vi "Microscope.Initialized.vi"(8 "error in (no error)":errorcluster, 10 "Initialized":T1, 11 "Microscope":refnum<class "Microscope.lvclass">) -> (0 "error out":errorcluster, 3 "Microscope out":refnum<class "Microscope.lvclass">)   [LabVIEW 2013, in "Microscope.lvclass"]
doc: "---------------------------------------------------------------\nJKI State Machine Objects™\nhttp://jki.net/state-machine-objects/\nCopyright (C) 2005-2015, JKI <info@jki.net>\nALL RIGHTS RESERVEDJKI State Machine Objects (SMO) 1.0.0.4\nJKI - JKI\nCopyright (c) 2015, JKI"
uses:
  Microscope.lvclass
  Typedefs/PublicEvents--Microscope.Initialized.ctl
panel:
  # "For instructions on how to use the JKI State Machine Objects, examples and video tutorials, visit:\nhttp://jki.net/state-machine-objects/\n\nJKI State Machine Objects™\nhttp://jki.net/state-machine-objects/\nCopyright (C) 2005-2015, JKI <info@jki.net>\nALL RIGHTS RESERVED"
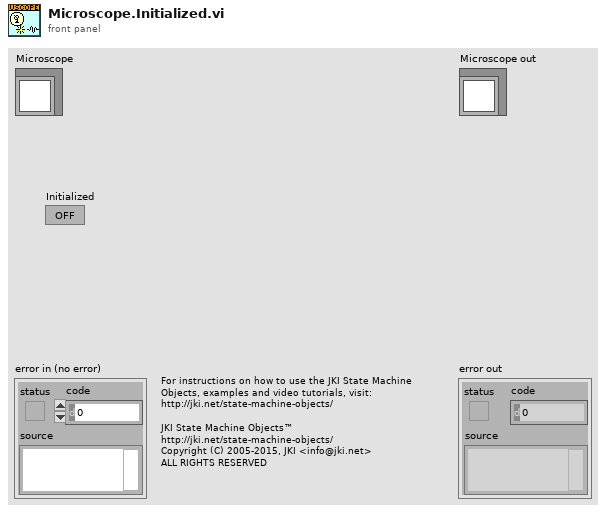
[diagram p1: front panel]
types:
  T1 = typedef "Microscope.lvclass/PublicEvents--Microscope.Initialized.ctl" = bool
  T2 = typedef "Microscope.lvclass/PrivateData--Ref.ctl" = refnum<data-value>
  T3 = typedef "Microscope.lvclass/PrivateData--Cluster.ctl" = cluster{"Public Events":T4, "Protected Events":T5, "Private Events":T6, "Dependencies":T7, "Configuration":T8}
  T4 = typedef "Microscope.lvclass/PublicEvents--Cluster.ctl" = cluster{"Value Changed":refnum<user-event>, "Initialized":refnum<user-event>}
  T5 = typedef "Microscope.lvclass/ProtectedEvents--Cluster.ctl" = cluster{"placeholder":refnum<user-event>}
  T6 = typedef "Microscope.lvclass/PrivateEvents--Cluster.ctl" = cluster{"New Value":refnum<user-event>, "Initialize":refnum<user-event>, "CaptureImageAtPosition":refnum<user-event>}
  T7 = typedef "Microscope.lvclass/Dependencies--Cluster.ctl" = cluster{"XYStage":refnum<class "XYStage.lvclass">, "Camera":refnum<class "Camera.lvclass">}
  T8 = typedef "Microscope.lvclass/Configuration--Cluster.ctl" = cluster{"XY Stage":string, "Camera":string, "image output folder":path, "filetype":string}
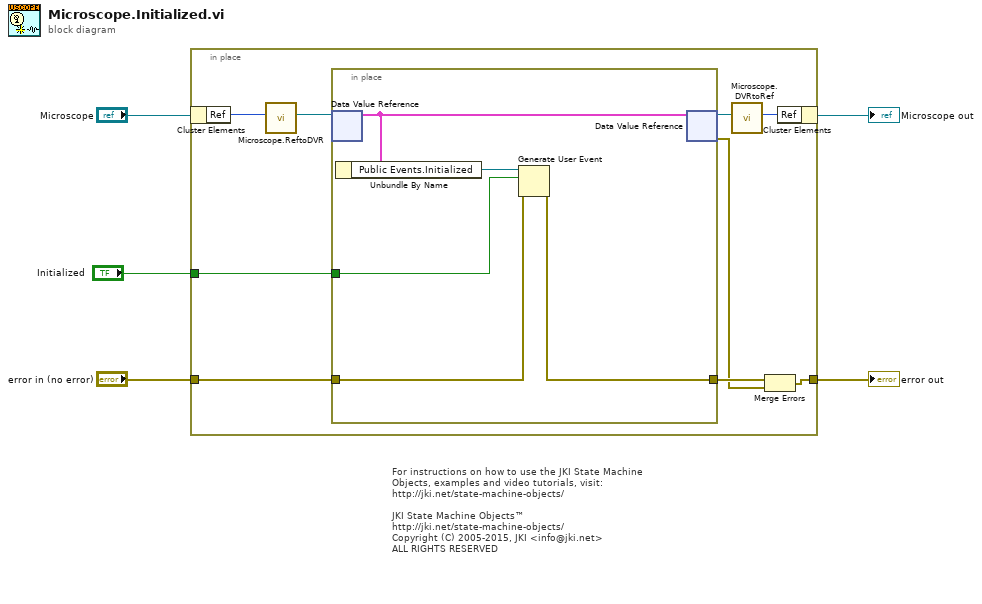
[diagram p0: block diagram]
diagram:
  # "For instructions on how to use the JKI State Machine Objects, examples and video tutorials, visit:\nhttp://jki.net/state-machine-objects/\n\nJKI State Machine Objects™\nhttp://jki.net/state-machine-objects/\nCopyright (C) 2005-2015, JKI <info@jki.net>\nALL RIGHTS RESERVED"
  n1 = in-place {
    in-place-border: "error in (no error)" -> [w14]
    in-place-border: [w11] -> w4
    in-place-border: "Initialized" -> [w8]
    n2 = in-place-cluster #1("Microscope") -> ("Ref"=w10:u32)
    n3 = call "Microscope.ReftoDVR.vi"("Ref"=w10) -> ("Ref"=w7:T2)  [unwired: 10 in]
    n4 = in-place {
      in-place-border: w14 -> [w17]
      in-place-border: [w16] -> w13
      in-place-border: w8 -> [w15]
      n5 = in-place-dvr #2(w7) -> (w19:T3)  [unwired: 1 out]
      n6 = Unbundle By Name(w19) -> ("Public Events.Initialized"=w18:refnum<user-event>)
      n7 = Generate User Event(user event=w18, event data cluster=w15, error in=w17) -> (error out=w16:errorcluster)  [unwired: 1 in, 1 out]
      n8 = in-place-dvr #2(w19) -> (w9:T2, w12:errorcluster)
    }
    n9 = call "Microscope.DVRtoRef.vi"("Ref"=w9) -> ("Ref"=w6:u32)  [unwired: 10 in]
    n10 = Merge Errors(w13, w12) -> (w11:errorcluster)
    n11 = in-place-cluster #1("Ref"=w6) -> (→"Microscope out":refnum<class "Microscope.lvclass">)
  }
  "error out" <- w4
